vi "Example WhileLoop ForLoop.vi"(8 "Error In":errorcluster, 11 "Boolean":bool) -> (0 "Error Out":errorcluster)   [LabVIEW 2014]
doc: "Testing VI contains WhileLoop and som operations inside and some other constants and functions for numbers used inside WhileLoop. Just for example parsing."
uses:
  <vilib>/measure/NI_MABase.lvlib
panel:
  out "signal out 2":waveform(dbl)
  out "signal out":waveform(dbl)
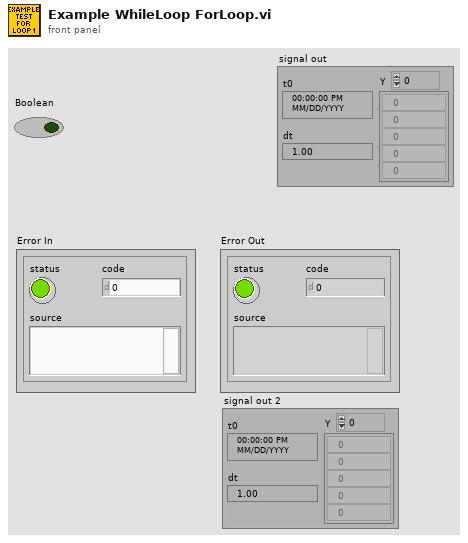
[diagram p1: front panel]
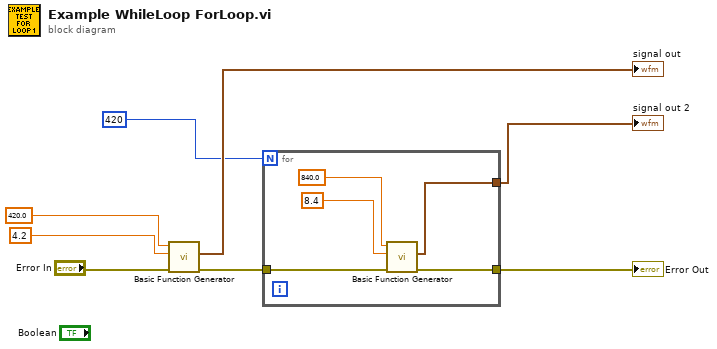
[diagram p0: block diagram]
diagram:
  n1 = call <vilib>:"Basic Function Generator.vi"("error in (no error)"="Error In", "amplitude"=4.2, "frequency"=420.0) -> ("error out"=w7:errorcluster, "signal out"=→"signal out":waveform(dbl))  [unwired: 6 in, 1 out]
  n2 = for {
    N: 420 -> [_]
    tunnel: [w9] -> w3
    tunnel: w7 -> [w13]
    tunnel: [w12] -> w1
    n3 = call <vilib>:"Basic Function Generator.vi"("error in (no error)"=w13, "amplitude"=8.4, "frequency"=840.0) -> ("error out"=w12:errorcluster, "signal out"=w9:waveform(dbl))  [unwired: 6 in, 1 out]
  }
  "Error Out" <- w1
  "signal out 2" <- w3
